vi "SignalConversion.vi"(6 "Reinitialize time? (F)":bool, 7 "Stop condition":T8={"Upper limit"={"Fz [pN]"=100000000.0, "Zext [nm]"=100000000.0, "Tau [pNnm]"=100000000.0, "Turn"=100000000.0, "Fx [pN]"=100000000.0, "Xext [nm]"=100000000.0, "Fy [pN]"=100000000.0, "Yext [nm]"=100000000.0, "time [s]"=100000000.0, "Delta Z signal"=100000000.0, "Delta Z bead [nm]"=100000000.0, "Z bead [nm]"=100000000.0, "Delta TrapZ [nm]"=100000000.0, "Delta Xsignal"=100000000.0, "X bead [nm]"=100000000.0, "Delta Ysignal"=100000000.0, "Y bead [nm]"=100000000.0, "Stop Condition"=100000000.0}, "Lower limit"={"Fz [pN]"=-100000000.0, "Zext [nm]"=-100000000.0, "Tau [pNnm]"=-100000000.0, "Turn"=-100000000.0, "Fx [pN]"=-100000000.0, "Xext [nm]"=-100000000.0, "Fy [pN]"=-100000000.0, "Yext [nm]"=-100000000.0, "time [s]"=-100000000.0, "Delta Z signal"=-100000000.0, "Delta Z bead [nm]"=-100000000.0, "Z bead [nm]"=-100000000.0, "Delta TrapZ [nm]"=-100000000.0, "Delta Xsignal"=-100000000.0, "X bead [nm]"=-100000000.0, "Delta Ysignal"=-100000000.0, "Y bead [nm]"=-100000000.0, "Stop Condition"=-100000000.0}}, 8 "error in (no error)":errorcluster, 9 "All data after scaling":T2, 10 "All DAQ channels":T1, 11 "Params in":T10={"TaskIDs"={"DAQ tasks"={"Px taskID"=0, "Py taskID"=0, "Pz taskID"=0, "AOM taskID"=0, "Clock taskID"=0, "AI taskID"=0}, "DVEHandle"=refnum}, "Manual Control"={"Rotation Control"={"Phase"=0.0, "A amp (0-120)"=75.0, "B amp (0-120)"=53.3, "mean freq  [MHz]\ndefault 39.99"=40.0, "freq difference [Hz]"=2.0, "Enable A"=TRUE, "Enable B"=TRUE}, "X piezo\n [nm]"=0.0, "Y peizo\n [nm]"=0.0, "trap height\n [nm]"=5.012658227848101, "AOM0 \nPower"=0.2}, "Piezo Calibr"={"Px2Vx(AO)"=nan, "Py2Vy(AO)"=nan, "Pz2Vz(AO)"=nan, "Min Px"=nan, "Min Py"=nan, "Min Pz"=nan, "Max Px"=nan, "Max Py"=nan, "Max Pz"=nan, "Vx0 (V)"=nan, "Vy0 (V)"=nan, "Vz0 (V)"=nan}, "Instrument Calibr"={"Angular compensation coeffs"=[], "TetherCenter"={"TrapX_AO 0 [nm]"=nan, "TrapY_AO 0 [nm]"=nan, "TrapZ_AO 0 [nm]"=nan}, "XYZsignal baseline"={"Xsignal0"=nan, "Ysignal0"=nan, "Zsignal0"=nan, "Zsig slope"=nan, "Z bead0"=nan}, "S and P to Vs0"={"Vs0/P"=1.0, "Vs0/S"=1.0}, "Psi"=0.0, "ePS:eRL drift correlation"={"Interc P"=nan, "Slope P"=nan, "Interc S"=nan, "Slope S"=nan}, "Current piezo volt AO"={"Vpx_AO [V]"=nan, "Vpy_AO [V]"=nan, "Vpz_AO [V]"=nan}}, "Cylinder Calibr"={"ZStiff"=nan, "Zsens"=nan, "AngStiff"=nan, "XStiff"=nan, "Xsens"=nan, "MaxEllip"=nan, "YStiff"=nan, "Ysens"=nan, "FocalShift"=nan, "Sfz"=nan, "1/Sz"=nan, "Stau"=nan, "Sfx"=nan, "1/Sx"=nan, "1/Sang"=nan, "Sfy"=nan, "1/Sy"=nan, "1/focal"=nan, "ZsignalHeightDependence (1/nm)"=0.0}, "DAQParams"={"Buffer size"=nan, "Scanning rate"=nan, "Average"=nan, "Sampling rate"=nan, "set dt"=nan}, "DAQ channel offsets"={"A0 [V]"=0.0, "D0 [V]"=0.0, "P0  [V]"=0.0, "S0 [V]"=0.0, "L0 [V]"=0.0, "R0 [V]"=0.0, "Vpx0 [V]"=0.0, "Vpy0 [V]"=0.0, "Vpz0 [V]"=0.0, "Vsum0 [V]"=0.0, "Vpx_AO0 [V]"=0.0, "Vpy_AO0 [V]"=0.0, "Vpz_AO0 [V]"=0.0}, "Z bead polynomial coeffs"=[nan, nan, nan, nan], "Skip button ref"=refnum, "z bead lookup table"={"z signal"=[], "z bead"=[]}, "SP->power Matrix"=[], "Ms2p"=[], "Mp2s"=[], "Polynomial coeff V_px,y,z 2 position (nm)"=[]} {"Cylinder Calibr"."ZsignalHeightDependence (1/nm)" format="%.4e"; "Instrument Calibr"."Psi" format="%#_2f"; "Manual Control"."Y peizo\n [nm]" step=100.0 scale=0.0..30000.0; "Manual Control"."AOM0 \nPower" scale=0.0..1.0; "Manual Control"."X piezo\n [nm]" step=100.0 scale=0.0..30000.0; "Manual Control"."Rotation Control"."mean freq  [MHz]\ndefault 39.99" min=0.0 step=0.01; "Manual Control"."Rotation Control"."B amp (0-120)" min=0.0 max=120.0 step=0.1 format="%.1f"; "Manual Control"."Rotation Control"."A amp (0-120)" min=0.0 max=120.0 step=0.1 format="%.1f"; "Manual Control"."Rotation Control"."Phase" scale=0.0..360.0; "Manual Control"."trap height\n [nm]" scale=1000.0..7500.0; "TaskIDs"."DAQ tasks"."Px taskID" format="%x"; "TaskIDs"."DAQ tasks"."Py taskID" format="%x"; "TaskIDs"."DAQ tasks"."Pz taskID" format="%x"; "TaskIDs"."DAQ tasks"."AOM taskID" format="%x"; "TaskIDs"."DAQ tasks"."Clock taskID" format="%x"; "TaskIDs"."DAQ tasks"."AI taskID" format="%x"}) -> (0 "error out":errorcluster, 2 "Physical Quantities cluster out":T9, 3 "Params out":T10={"TaskIDs"={"DAQ tasks"={"Px taskID"=0, "Py taskID"=0, "Pz taskID"=0, "AOM taskID"=0, "Clock taskID"=0, "AI taskID"=0}, "DVEHandle"=refnum}, "Manual Control"={"Rotation Control"={"Phase"=0.0, "A amp (0-120)"=75.0, "B amp (0-120)"=53.3, "mean freq  [MHz]\ndefault 39.99"=40.0, "freq difference [Hz]"=2.0, "Enable A"=TRUE, "Enable B"=TRUE}, "X piezo\n [nm]"=0.0, "Y peizo\n [nm]"=0.0, "trap height\n [nm]"=5.012658227848101, "AOM0 \nPower"=0.2}, "Piezo Calibr"={"Px2Vx(AO)"=nan, "Py2Vy(AO)"=nan, "Pz2Vz(AO)"=nan, "Min Px"=nan, "Min Py"=nan, "Min Pz"=nan, "Max Px"=nan, "Max Py"=nan, "Max Pz"=nan, "Vx0 (V)"=nan, "Vy0 (V)"=nan, "Vz0 (V)"=nan}, "Instrument Calibr"={"Angular compensation coeffs"=[], "TetherCenter"={"TrapX_AO 0 [nm]"=nan, "TrapY_AO 0 [nm]"=nan, "TrapZ_AO 0 [nm]"=nan}, "XYZsignal baseline"={"Xsignal0"=nan, "Ysignal0"=nan, "Zsignal0"=nan, "Zsig slope"=nan, "Z bead0"=nan}, "S and P to Vs0"={"Vs0/P"=1.0, "Vs0/S"=1.0}, "Psi"=0.0, "ePS:eRL drift correlation"={"Interc P"=nan, "Slope P"=nan, "Interc S"=nan, "Slope S"=nan}, "Current piezo volt AO"={"Vpx_AO [V]"=nan, "Vpy_AO [V]"=nan, "Vpz_AO [V]"=nan}}, "Cylinder Calibr"={"ZStiff"=nan, "Zsens"=nan, "AngStiff"=nan, "XStiff"=nan, "Xsens"=nan, "MaxEllip"=nan, "YStiff"=nan, "Ysens"=nan, "FocalShift"=nan, "Sfz"=nan, "1/Sz"=nan, "Stau"=nan, "Sfx"=nan, "1/Sx"=nan, "1/Sang"=nan, "Sfy"=nan, "1/Sy"=nan, "1/focal"=nan, "ZsignalHeightDependence (1/nm)"=0.0}, "DAQParams"={"Buffer size"=nan, "Scanning rate"=nan, "Average"=nan, "Sampling rate"=nan, "set dt"=nan}, "DAQ channel offsets"={"A0 [V]"=0.0, "D0 [V]"=0.0, "P0  [V]"=0.0, "S0 [V]"=0.0, "L0 [V]"=0.0, "R0 [V]"=0.0, "Vpx0 [V]"=0.0, "Vpy0 [V]"=0.0, "Vpz0 [V]"=0.0, "Vsum0 [V]"=0.0, "Vpx_AO0 [V]"=0.0, "Vpy_AO0 [V]"=0.0, "Vpz_AO0 [V]"=0.0}, "Z bead polynomial coeffs"=[nan, nan, nan, nan], "Skip button ref"=refnum, "z bead lookup table"={"z signal"=[], "z bead"=[]}, "SP->power Matrix"=[], "Ms2p"=[], "Mp2s"=[], "Polynomial coeff V_px,y,z 2 position (nm)"=[]} {"Cylinder Calibr"."ZsignalHeightDependence (1/nm)" format="%.4e"; "Instrument Calibr"."Psi" format="%#_2f"; "Manual Control"."Y peizo\n [nm]" step=100.0 scale=0.0..30000.0; "Manual Control"."AOM0 \nPower" scale=0.0..1.0; "Manual Control"."X piezo\n [nm]" step=100.0 scale=0.0..30000.0; "Manual Control"."Rotation Control"."mean freq  [MHz]\ndefault 39.99" min=0.0 step=0.01; "Manual Control"."Rotation Control"."B amp (0-120)" min=0.0 max=120.0 step=0.1 format="%.1f"; "Manual Control"."Rotation Control"."A amp (0-120)" min=0.0 max=120.0 step=0.1 format="%.1f"; "Manual Control"."Rotation Control"."Phase" scale=0.0..360.0; "Manual Control"."trap height\n [nm]" scale=1000.0..7500.0; "TaskIDs"."DAQ tasks"."Px taskID" format="%x"; "TaskIDs"."DAQ tasks"."Py taskID" format="%x"; "TaskIDs"."DAQ tasks"."Pz taskID" format="%x"; "TaskIDs"."DAQ tasks"."AOM taskID" format="%x"; "TaskIDs"."DAQ tasks"."Clock taskID" format="%x"; "TaskIDs"."DAQ tasks"."AI taskID" format="%x"}, 4 "In range and \"skip\" button is off?":bool, 5 "Code Signal out of Range":u32)   [LabVIEW 2020, in "SignalConverson.lvlib"]
uses:
  SignalConverson.lvlib
  Initialization/Param.ctl
  Initialization/ManualCtrl.ctl
  Initialization/DVESetting.ctl
  Initialization/CylinderCalibrNew.ctl
  DAQChannelOffsets.ctl
  <vilib>/Analysis/Matrix/Datatypes/RealMatrix.ctl
  Initialization/Physical Quantitites.ctl
  StopCondition.ctl
  ScaledData.ctl
  Measrured TrapXYZ.ctl
  Data Before Angle Compensation.ctl
  Angle compensated data.ctl
  XYZ Signals.ctl
  Set TrapXYZ.ctl
  DAQChannelRawData.ctl
  <vilib>/Analysis/polynomials.llb/Scalar Polynomial Evaluation (DBL).vi
  <vilib>/Analysis/NI_AALPro.lvlib
  Initialization/Initialization.lvlib
  <vilib>/Analysis/Matrix/NI_Matrix.lvlib
panel:
  in  "Method for Zbead calculation (hard coded)":u16(ring) items=["Linear", "Polynomial", "Lookup table"]
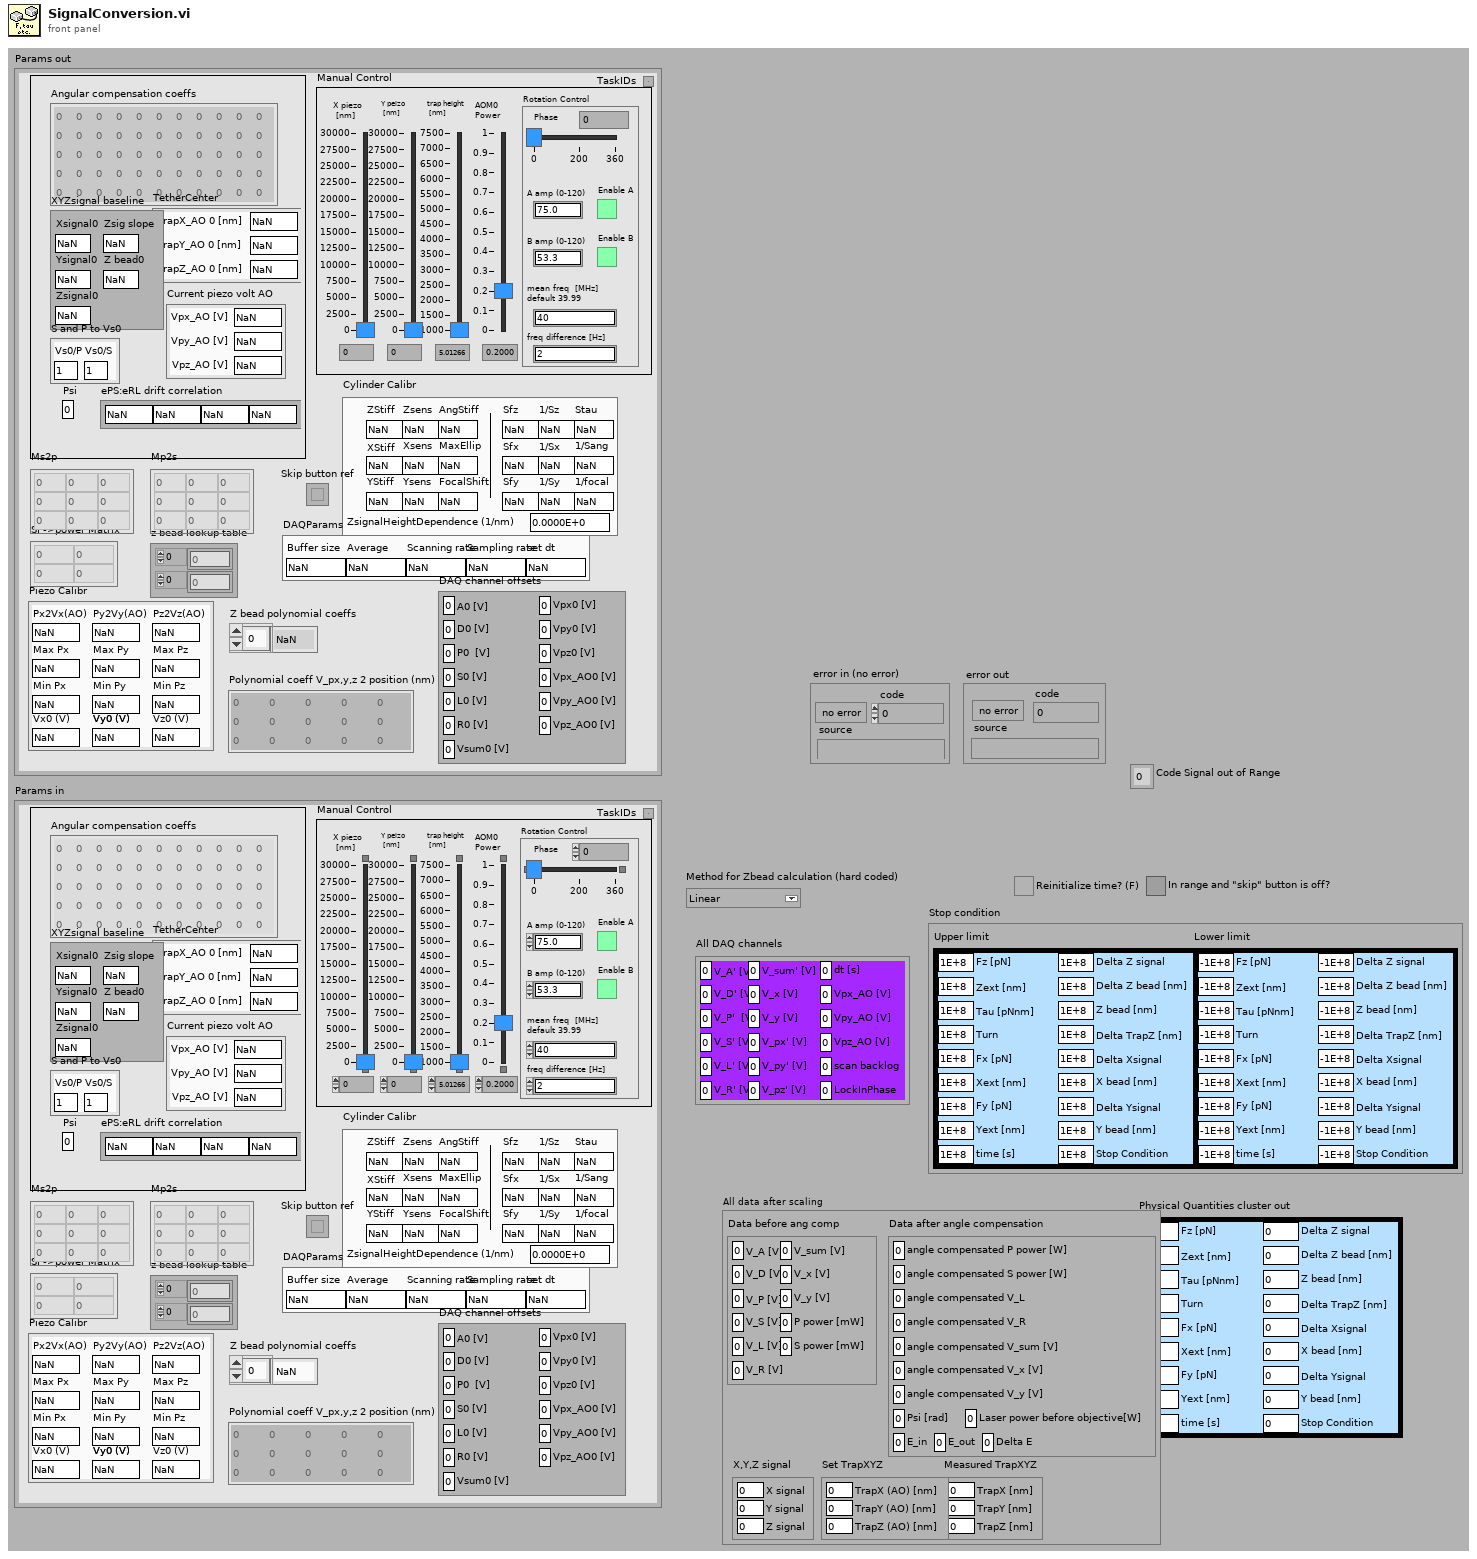
[diagram p1: front panel]
types:
  T1 = typedef "SignalConverson.lvlib/DAQChannelRawData.ctl" = cluster{"V_A' [V]":dbl, "V_D' [V]":dbl, "V_P'  [V]":dbl, "V_S' [V]":dbl, "V_L' [V]":dbl, "V_R' [V]":dbl, "V_sum' [V]":dbl, "V_x [V]":dbl, "V_y [V]":dbl, "V_px' [V]":dbl, "V_py' [V]":dbl, "V_pz' [V]":dbl, "dt [s]":dbl, "Vpx_AO [V]":dbl, "Vpy_AO [V]":dbl, "Vpz_AO [V]":dbl, "scan backlog":u32, "LockInPhase":dbl}
  T2 = typedef "SignalConverson.lvlib/ScaledData.ctl" = cluster{"Measured TrapXYZ":T3, "Data before ang comp":T4, "Data after angle compensation":T5, "X,Y,Z signal":T6, "Set TrapXYZ":T7}
  T3 = typedef "SignalConverson.lvlib/Measrured TrapXYZ.ctl" = cluster{"TrapX [nm]":dbl, "TrapY [nm]":dbl, "TrapZ [nm]":dbl}
  T4 = typedef "SignalConverson.lvlib/Data Before Angle Compensation.ctl" = cluster{"V_A [V]":dbl, "V_D [V]":dbl, "V_P [V]":dbl, "V_S [V]":dbl, "V_L [V]":dbl, "V_R [V]":dbl, "V_sum [V]":dbl, "V_x [V]":dbl, "V_y [V]":dbl, "P power [mW]":dbl, "S power [mW]":dbl}
  T5 = typedef "SignalConverson.lvlib/Angle compensated data.ctl" = cluster{"angle compensated P power [W]":dbl, "angle compensated S power [W]":dbl, "angle compensated V_L":dbl, "angle compensated V_R":dbl, "angle compensated V_sum [V]":dbl, "angle compensated V_x [V]":dbl, "angle compensated V_y [V]":dbl, "Psi [rad]":dbl, "Laser power before objective[W]":dbl, "E_in":dbl, "E_out":dbl, "Delta E":dbl}
  T6 = typedef "SignalConverson.lvlib/XYZ Signals.ctl" = cluster{"X signal":dbl, "Y signal":dbl, "Z signal":dbl}
  T7 = typedef "SignalConverson.lvlib/Set TrapXYZ.ctl" = cluster{"TrapX (AO) [nm]":dbl, "TrapY (AO) [nm]":dbl, "TrapZ (AO) [nm]":dbl}
  T8 = typedef "SignalConverson.lvlib/StopCondition.ctl" = cluster{"Upper limit":T9, "Lower limit":T9}
  T9 = typedef "SignalConverson.lvlib/Physical Quantitites.ctl" = cluster{"Fz [pN]":dbl, "Zext [nm]":dbl, "Tau [pNnm]":dbl, "Turn":dbl, "Fx [pN]":dbl, "Xext [nm]":dbl, "Fy [pN]":dbl, "Yext [nm]":dbl, "time [s]":dbl, "Delta Z signal":dbl, "Delta Z bead [nm]":dbl, "Z bead [nm]":dbl, "Delta TrapZ [nm]":dbl, "Delta Xsignal":dbl, "X bead [nm]":dbl, "Delta Ysignal":dbl, "Y bead [nm]":dbl, "Stop Condition":dbl}
  T10 = typedef "Initialization.lvlib/Param.ctl" = cluster{"TaskIDs":cluster{"DAQ tasks":cluster{"Px taskID":u32, "Py taskID":u32, "Pz taskID":u32, "AOM taskID":u32, "Clock taskID":u32, "AI taskID":u32}, "DVEHandle":refnum<file>}, "Manual Control":T11, "Piezo Calibr":cluster{"Px2Vx(AO)":dbl, "Py2Vy(AO)":dbl, "Pz2Vz(AO)":dbl, "Min Px":dbl, "Min Py":dbl, "Min Pz":dbl, "Max Px":dbl, "Max Py":dbl, "Max Pz":dbl, "Vx0 (V)":dbl, "Vy0 (V)":dbl, "Vz0 (V)":dbl}, "Instrument Calibr":cluster{"Angular compensation coeffs":dbl[][], "TetherCenter":cluster{"TrapX_AO 0 [nm]":dbl, "TrapY_AO 0 [nm]":dbl, "TrapZ_AO 0 [nm]":dbl}, "XYZsignal baseline":cluster{"Xsignal0":dbl, "Ysignal0":dbl, "Zsignal0":dbl, "Zsig slope":dbl, "Z bead0":dbl}, "S and P to Vs0":cluster{"Vs0/P":dbl, "Vs0/S":dbl}, "Psi":dbl, "ePS:eRL drift correlation":cluster{"Interc P":dbl, "Slope P":dbl, "Interc S":dbl, "Slope S":dbl}, "Current piezo volt AO":cluster{"Vpx_AO [V]":dbl, "Vpy_AO [V]":dbl, "Vpz_AO [V]":dbl}}, "Cylinder Calibr":T13, "DAQParams":cluster{"Buffer size":dbl, "Scanning rate":dbl, "Average":dbl, "Sampling rate":dbl, "set dt":dbl}, "DAQ channel offsets":T14, "Z bead polynomial coeffs":dbl[], "Skip button ref":refnum<vi>, "z bead lookup table":cluster{"z signal":dbl[], "z bead":dbl[]}, "SP->power Matrix":T15, "Ms2p":T15, "Mp2s":T15, "Polynomial coeff V_px,y,z 2 position (nm)":dbl[][]}
  T11 = typedef "Initialization.lvlib/ManualCtrl.ctl" = cluster{"Rotation Control":T12, "X piezo\n [nm]":dbl, "Y peizo\n [nm]":dbl, "trap height\n [nm]":dbl, "AOM0 \nPower":dbl}
  T12 = typedef "Initialization.lvlib/DVESetting.ctl" = cluster{"Phase":dbl, "A amp (0-120)":dbl, "B amp (0-120)":dbl, "mean freq  [MHz]\ndefault 39.99":dbl, "freq difference [Hz]":dbl, "Enable A":bool, "Enable B":bool}
  T13 = typedef "Initialization.lvlib/CylinderCalibrNew.ctl" = cluster{"ZStiff":dbl, "Zsens":dbl, "AngStiff":dbl, "XStiff":dbl, "Xsens":dbl, "MaxEllip":dbl, "YStiff":dbl, "Ysens":dbl, "FocalShift":dbl, "Sfz":dbl, "1/Sz":dbl, "Stau":dbl, "Sfx":dbl, "1/Sx":dbl, "1/Sang":dbl, "Sfy":dbl, "1/Sy":dbl, "1/focal":dbl, "ZsignalHeightDependence (1/nm)":dbl}
  T14 = typedef "SignalConverson.lvlib/DAQChannelOffsets.ctl" = cluster{"A0 [V]":dbl, "D0 [V]":dbl, "P0  [V]":dbl, "S0 [V]":dbl, "L0 [V]":dbl, "R0 [V]":dbl, "Vpx0 [V]":dbl, "Vpy0 [V]":dbl, "Vpz0 [V]":dbl, "Vsum0 [V]":dbl, "Vpx_AO0 [V]":dbl, "Vpy_AO0 [V]":dbl, "Vpz_AO0 [V]":dbl}
  T15 = typedef "NI_Matrix.lvlib/RealMatrix.ctl" = dbl[][]
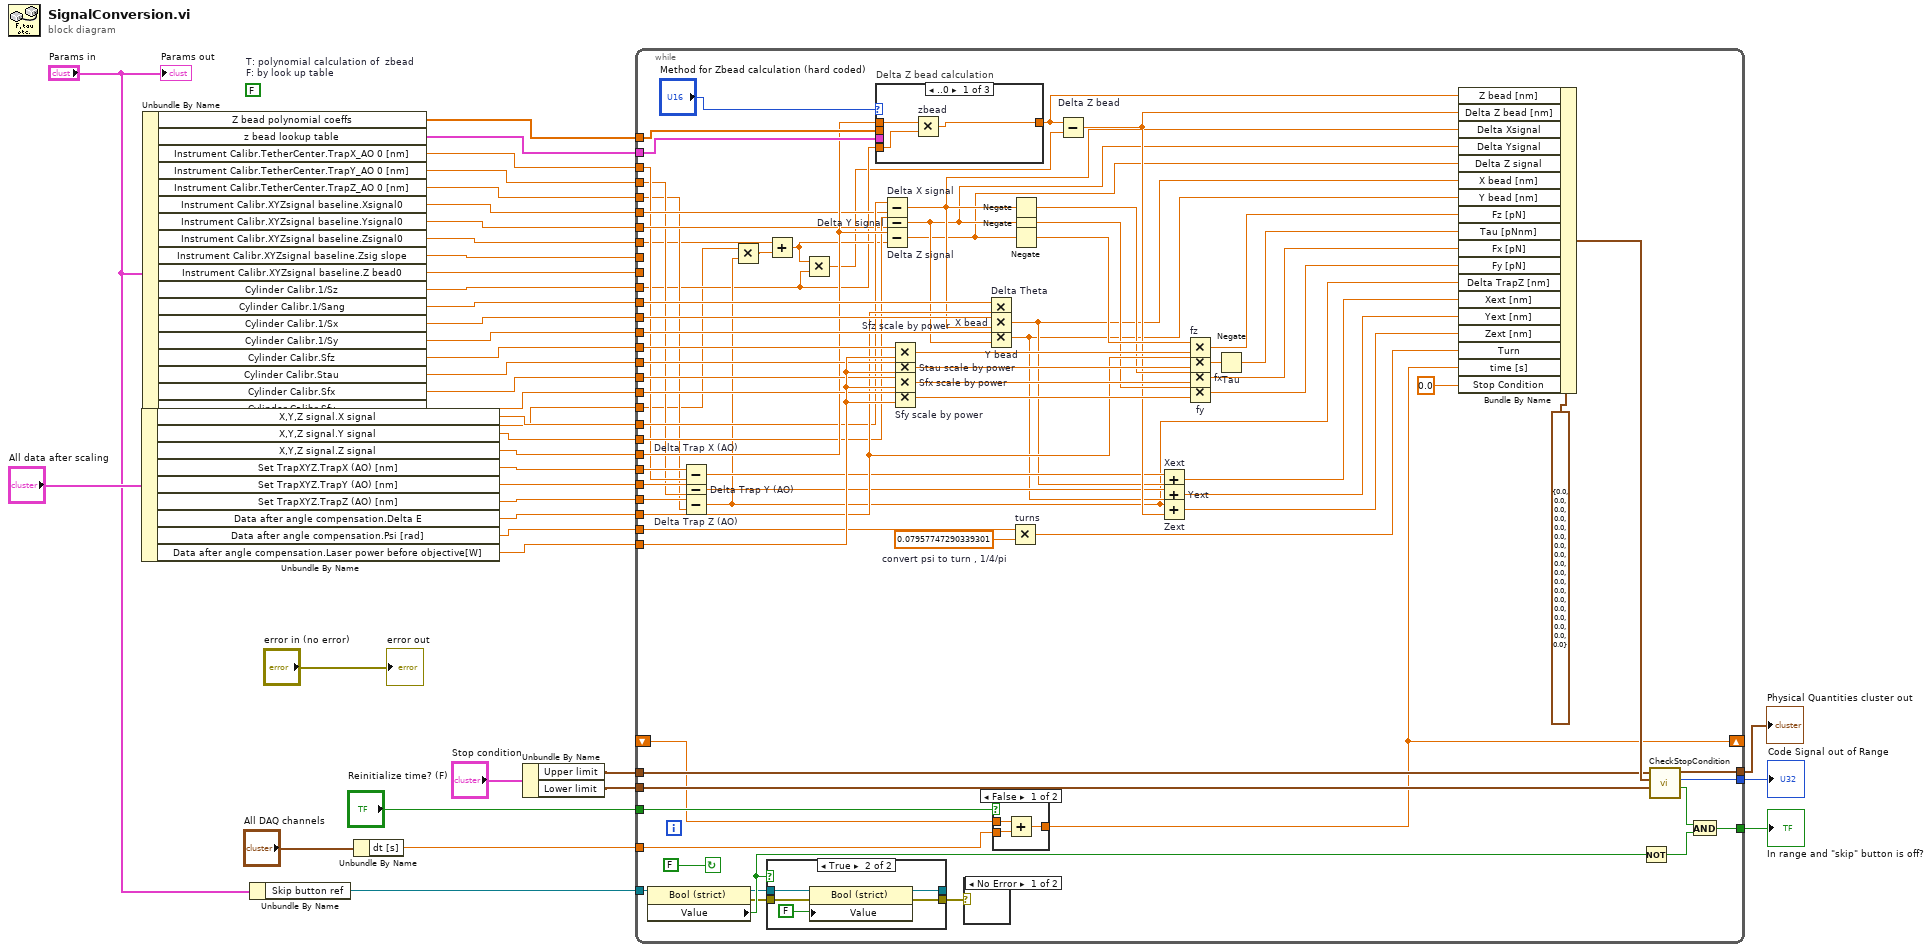
[diagram p0: block diagram]
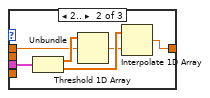
[diagram p2: hidden frame]
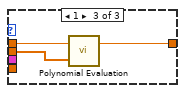
[diagram p3: hidden frame]
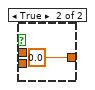
[diagram p6: hidden frame]
diagram:
  (unwired) FALSE  # T: polynomial calculation of  zbead F: by look up table
  n1 = Unbundle By Name("All data after scaling") -> ("X,Y,Z signal.X signal"=w30:dbl, "X,Y,Z signal.Y signal"=w31:dbl, "X,Y,Z signal.Z signal"=w32:dbl, "Set TrapXYZ.TrapX (AO) [nm]"=w29:dbl, "Set TrapXYZ.TrapY (AO) [nm]"=w28:dbl, "Set TrapXYZ.TrapZ (AO) [nm]"=w27:dbl, "Data after angle compensation.Delta E"=w26:dbl, "Data after angle compensation.Psi [rad]"=w25:dbl, "Data after angle compensation.Laser power before objective[W]"=w22:dbl)
  n2 = Unbundle By Name("Params in") -> ("Z bead polynomial coeffs"=w35:dbl[], "z bead lookup table"=w34:cluster{"z signal":dbl[], "z bead":dbl[]}, "Instrument Calibr.TetherCenter.TrapX_AO 0 [nm]"=w21:dbl, "Instrument Calibr.TetherCenter.TrapY_AO 0 [nm]"=w20:dbl, "Instrument Calibr.TetherCenter.TrapZ_AO 0 [nm]"=w19:dbl, "Instrument Calibr.XYZsignal baseline.Xsignal0"=w18:dbl, "Instrument Calibr.XYZsignal baseline.Ysignal0"=w17:dbl, "Instrument Calibr.XYZsignal baseline.Zsignal0"=w16:dbl, "Instrument Calibr.XYZsignal baseline.Zsig slope"=w15:dbl, "Instrument Calibr.XYZsignal baseline.Z bead0"=w14:dbl, "Cylinder Calibr.1/Sz"=w13:dbl, "Cylinder Calibr.1/Sang"=w12:dbl, "Cylinder Calibr.1/Sx"=w11:dbl, "Cylinder Calibr.1/Sy"=w10:dbl, "Cylinder Calibr.Sfz"=w9:dbl, "Cylinder Calibr.Stau"=w8:dbl, "Cylinder Calibr.Sfx"=w7:dbl, "Cylinder Calibr.Sfy"=w6:dbl, "Cylinder Calibr.ZsignalHeightDependence (1/nm)"=w1:dbl)
  n3 = Unbundle By Name("Params in") -> ("Skip button ref"=w5:refnum<vi>)
  n4 = Unbundle By Name("All DAQ channels") -> ("dt [s]"=w23:dbl)
  n5 = Unbundle By Name("Stop condition") -> ("Upper limit"=w38:T9, "Lower limit"=w37:T9)
  n6 = while {
    tunnel: [w95] -> w40
    tunnel: [w110] -> w41
    tunnel: w38 -> [w117]
    tunnel: w37 -> [w116]
    tunnel: "Reinitialize time? (F)" -> [w114]
    shift-right: [w56] -> _
    shift-left: _ -> [w113]
    tunnel: w35 -> [w104]
    tunnel: w34 -> [w105]
    tunnel: w32 -> [w90]
    tunnel: w31 -> [w83]
    tunnel: w30 -> [w82]
    tunnel: w29 -> [w73]
    tunnel: w28 -> [w72]
    tunnel: w27 -> [w71]
    tunnel: w26 -> [w84]
    tunnel: w25 -> [w78]
    tunnel: w23 -> [w100]
    tunnel: w22 -> [w103]
    tunnel: w21 -> [w70]
    tunnel: w20 -> [w69]
    tunnel: w19 -> [w68]
    tunnel: w18 -> [w80]
    tunnel: w17 -> [w81]
    tunnel: w16 -> [w47]
    tunnel: w15 -> [_]
    tunnel: w14 -> [_]
    tunnel: w13 -> [w44]
    tunnel: w12 -> [w93]
    tunnel: w11 -> [w92]
    tunnel: w10 -> [w91]
    tunnel: w9 -> [w96]
    tunnel: w8 -> [w97]
    tunnel: w7 -> [w98]
    tunnel: w6 -> [w99]
    tunnel: w5 -> [w102]
    tunnel: [w94] -> w3
    tunnel: w1 -> [w42]
    stop <- FALSE continue-if-true
    w79 = 0.07957747290339301  # convert psi to turn , 1/4/pi
    n7 = property class="Bool (strict)"(reference=w102) -> (reference out=w108:refnum<vi>, error out=w107:errorcluster, "Value"=w109:bool)  [unwired: 1 in]
    n8 = Subtract "Delta Trap X (AO)"(x=w73, y=w70) -> (x-y=w67:dbl)
    n9 = Subtract "Delta Trap Y (AO)"(x=w72, y=w69) -> (x-y=w66:dbl)
    n10 = Subtract "Delta Trap Z (AO)"(x=w71, y=w68) -> (x-y=w46:dbl)
    n11 = Multiply(x=w42, y=w46) -> (x*y=w48:dbl)
    n12 = Add(x=w47, y=w48) -> (x+y=w45:dbl)
    n13 = case shown="True" w109 {
      tunnel: w108 -> [w131 w136]
      tunnel: [w131 w134] -> _
      tunnel: w107 -> [_ w133]
      tunnel: [_ w132] -> w106
      frame False {
      }
      frame True {
        n14 = property class="Bool (strict)"(reference=w136, error in=w133, "Value"=FALSE) -> (reference out=w134:refnum<vi>, error out=w132:errorcluster)
      }
    }
    n15 = Multiply(x=w45, y=w44) -> (x*y=w43:dbl)
    n16 = case "Delta Z bead calculation" shown="..0" "Method for Zbead calculation (hard coded)" {
      tunnel: w104 -> [_ _ w130]
      tunnel: w90 -> [w121 w125 w129]
      tunnel: [w119 w122 w128] -> w75
      tunnel: w105 -> [_ w127 _]
      tunnel: w44 -> [w120 _ _]
      frame ..0 {
        n17 = Multiply "zbead"(x=w121, y=w120) -> (x*y=w119:dbl)
      }
      frame 2.. {
        n18 = Unbundle(w127) -> ("z signal"=w126:dbl[], "z bead"=w124:dbl[])
        n19 = Threshold 1D Array(2:w125, 3:w126) -> (0:w123:dbl)  [unwired: 1 in]
        n20 = Interpolate 1D Array(1:w123, 2:w124) -> (0:w122:dbl)
      }
      frame 1 {
        n21 = call-poly <vilib>:"Polynomial Evaluation.vi"("P(x)"=w130, "a"=w129) -> ("P(a)"=w128:dbl)  [unwired: 1 out]
      }
    }
    n22 = Subtract "Delta X signal"(x=w82, y=w80) -> (x-y=w65:dbl)
    n23 = Subtract "Delta Y signal"(x=w83, y=w81) -> (x-y=w64:dbl)
    n24 = Subtract "Delta Z signal"(x=w90, y=w45) -> (x-y=w63:dbl)
    n25 = Multiply "Sfz scale by power"(x=w96, y=w103) -> (x*y=w89:dbl)
    n26 = Multiply "Stau scale by power"(x=w97, y=w103) -> (x*y=w88:dbl)
    n27 = Multiply "Sfx scale by power"(x=w98, y=w103) -> (x*y=w87:dbl)
    n28 = Multiply "Sfy scale by power"(x=w99, y=w103) -> (x*y=w86:dbl)
    n29 = case shown="No Error" w106 {
      frame No Error {
      }
      frame Error {
      }
    }
    n30 = Multiply "Delta Theta"(x=w93, y=w84) -> ()  [unwired: 1 out]
    n31 = Multiply "X bead"(x=w92, y=w65) -> (x*y=w59:dbl)
    n32 = Multiply "Y bead"(x=w91, y=w64) -> (x*y=w58:dbl)
    n33 = case shown="False" w114 {
      tunnel: w113 -> [w138 _]
      tunnel: [w139 0.0] -> w56
      tunnel: w100 -> [w137 _]
      frame False {
        n34 = Add(x=w138, y=w137) -> (x+y=w139:dbl)
      }
      frame True {
      }
    }
    n35 = Multiply "turns"(x=w78, y=w79) -> (x*y=w55:dbl)
    n36 = Negate ("The direction of force and Z signal are opposite")(x=w65) -> (-x=w76:dbl)
    n37 = Negate ("The direction of force and Z signal are opposite")(x=w64) -> (-x=w77:dbl)
    n38 = Negate ("The direction of force and Z signal are opposite")(x=w63) -> (-x=w85:dbl)
    n39 = Subtract "Delta Z bead"(x=w75, y=w43) -> (x-y=w74:dbl)
    n40 = Add "Xext"(x=w67, y=w59) -> (x+y=w54:dbl)
    n41 = Add "Yext"(x=w66, y=w58) -> (x+y=w52:dbl)
    n42 = Add "Zext"(x=w46, y=w74) -> (x+y=w53:dbl)
    n43 = Multiply "fz"(x=w85, y=w89) -> (x*y=w62:dbl)
    n44 = Multiply(x=w84, y=w88) -> (x*y=w50:dbl)
    n45 = Multiply "fx"(x=w76, y=w87) -> (x*y=w61:dbl)
    n46 = Multiply "fy"(x=w77, y=w86) -> (x*y=w60:dbl)
    n47 = Negate "Tau"(x=w50) -> (-x=w49:dbl)
    n48 = Bundle By Name(cluster=T9 {"Fz [pN]"=0.0, "Zext [nm]"=0.0, "Tau [pNnm]"=0.0, "Turn"=0.0, "Fx [pN]"=0.0, "Xext [nm]"=0.0, "Fy [pN]"=0.0, "Yext [nm]"=0.0, "time [s]"=0.0, "Delta Z signal"=0.0, "Delta Z bead [nm]"=0.0, "Z bead [nm]"=0.0, "Delta TrapZ [nm]"=0.0, "Delta Xsignal"=0.0, "X bead [nm]"=0.0, "Delta Ysignal"=0.0, "Y bead [nm]"=0.0, "Stop Condition"=0.0} ("Physical Quantities cluster out"), "Z bead [nm]"=w75, "Delta Z bead [nm]"=w74, "Delta Xsignal"=w65, "Delta Ysignal"=w64, "Delta Z signal"=w63, "X bead [nm]"=w59, "Y bead [nm]"=w58, "Fz [pN]"=w62, "Tau [pNnm]"=w49, "Fx [pN]"=w61, "Fy [pN]"=w60, "Delta TrapZ [nm]"=w46, "Xext [nm]"=w54, "Yext [nm]"=w52, "Zext [nm]"=w53, "Turn"=w55, "time [s]"=w56, "Stop Condition"=0.0) -> (w118:T9)
    n49 = Not(x=w109) -> (.not. x?=w112:bool)
    n50 = call "CheckStopCondition.vi"("Lower limit"=w116, "Data"=w118, "Upper limit"=w117) -> ("In range?"=w111:bool, "Which Signal is out of Range?"=w95:u32, "Data out"=w94:T9)  [unwired: 2 in]
    n51 = And(x=w111, y=w112) -> (x .and. y?=w110:bool)
  }
  "Physical Quantities cluster out" <- w3
  "In range and \"skip\" button is off?" <- w41
  "Code Signal out of Range" <- w40
  "Params out" <- "Params in"
  "error out" <- "error in (no error)"
